vi "InitializeLineDigital.vi"(2 "Store Data":bool, 3 "Image Settings":T1={"Start Position (µm)"={"x"=0.0, "y"=0.0, "z"=0.0}, "End Position (µm)"={"x"=10.0, "y"=10.0, "z"=0.0}, "Image Resolution (nm/pixel)"={"x"=50.0, "y"=50.0, "z"=100.0}, "Image Size (µm)"={"x"=10.0, "y"=10.0, "z"=0.0}, "Image Size (pixel)"={"x"=50, "y"=50, "z"=0}, "Time Resolution\n(ms/pixel)"=7.0, "1st Axis"=0, "2nd Axis"=1, "Retrace"=FALSE, "Estimated Time"=""} {"2nd Axis" items=["x", "y", "z"]; "1st Axis" items=["x", "y", "z"]; "Time Resolution\n(ms/pixel)" format="%.2f"; "Image Resolution (nm/pixel)"."z" format="%.2f"; "Image Resolution (nm/pixel)"."y" format="%.2f"; "Image Resolution (nm/pixel)"."x" format="%.2f"; "Image Size (µm)"."z" format="%.2f"; "Image Size (µm)"."y" format="%.2f"; "Image Size (µm)"."x" format="%.2f"; "End Position (µm)"."z" format="%.2f"; "End Position (µm)"."y" format="%.2f"; "End Position (µm)"."x" format="%.2f"; "Start Position (µm)"."z" format="%.2f"; "Start Position (µm)"."y" format="%.2f"; "Start Position (µm)"."x" format="%.2f"}, 4 "error in (no error)":errorcluster, 5 "Destination:":path) -> (0 "error out":errorcluster, 1 "Busy":bool)   [LabVIEW 2009]
uses:
  ImageSettings.ctt
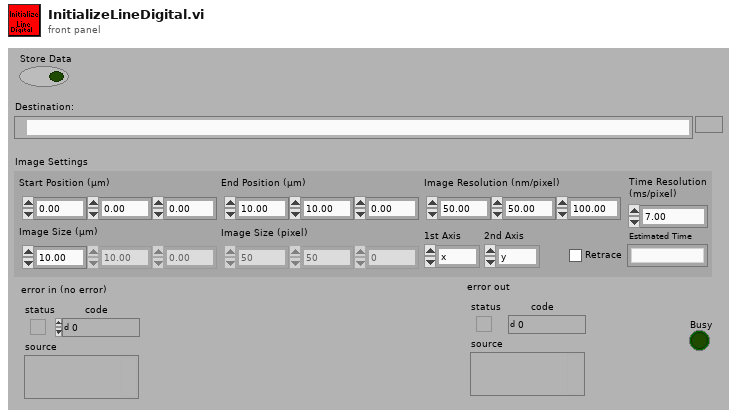
[diagram p1: front panel]
types:
  T1 = typedef "ImageSettings.ctt" = cluster{"Start Position (µm)":cluster{"x":dbl, "y":dbl, "z":dbl}, "End Position (µm)":cluster{"x":dbl, "y":dbl, "z":dbl}, "Image Resolution (nm/pixel)":cluster{"x":dbl, "y":dbl, "z":dbl}, "Image Size (µm)":cluster{"x":dbl, "y":dbl, "z":dbl}, "Image Size (pixel)":cluster{"x":u32, "y":u32, "z":u32}, "Time Resolution\n(ms/pixel)":dbl, "1st Axis":u16, "2nd Axis":u16, "Retrace":bool, "Estimated Time":string}
  T2 = typedef "LineScanStatus.ctt" = cluster{"in line":bool, "line status":cluster{"count":u32, "current":cluster{"x":u32, "y":u32, "z":u32}}, "plane status":cluster{"count":u32, "current":cluster{"x":u32, "y":u32, "z":u32}}, "new line step":cluster{"x":dbl, "y":dbl, "z":dbl}, "new plane step":cluster{"x":dbl, "y":dbl, "z":dbl}}
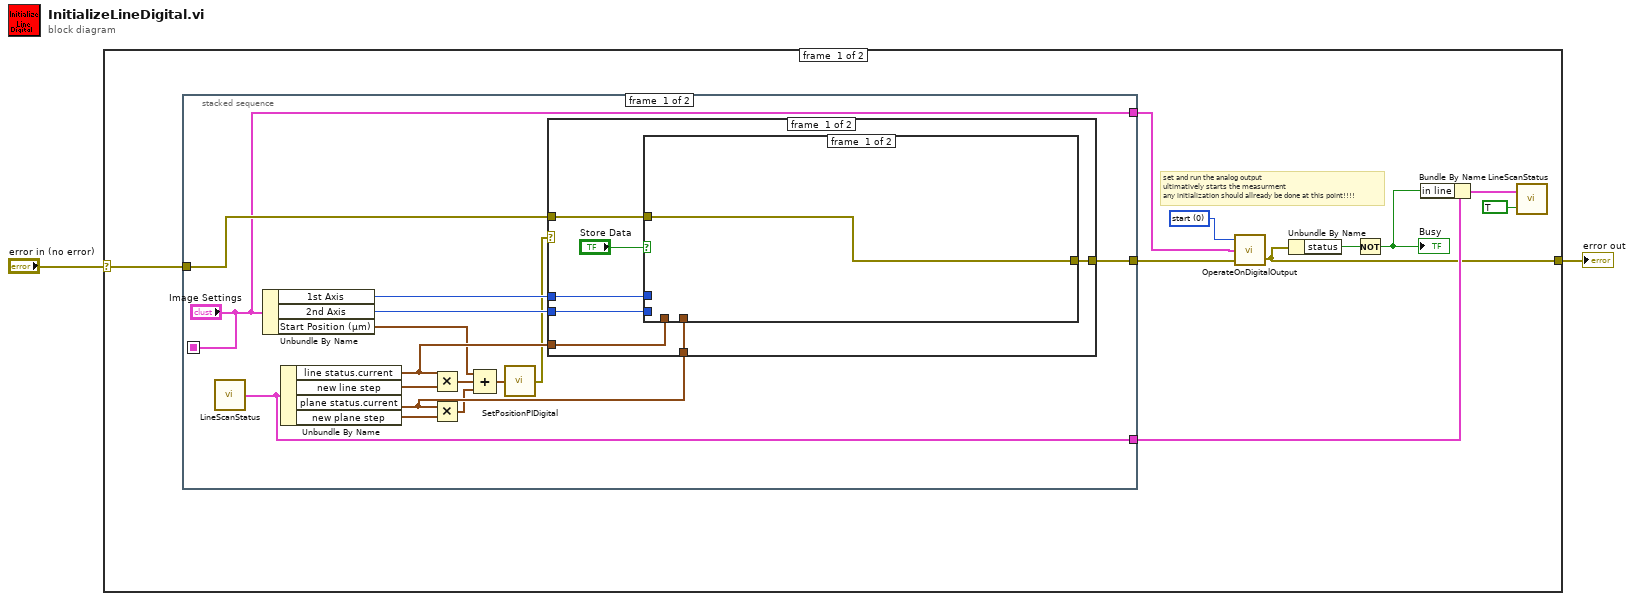
[diagram p0: block diagram]
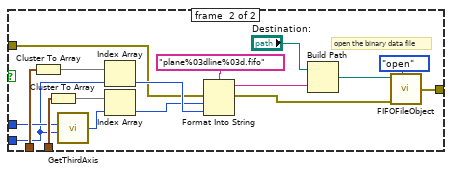
[diagram p2: hidden frame]
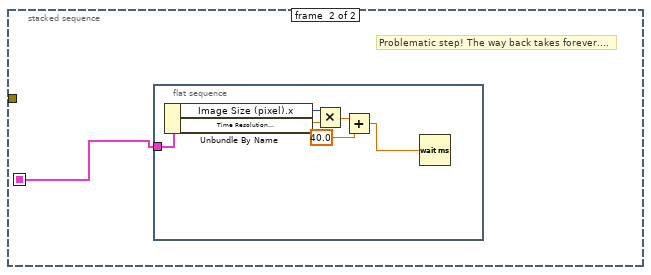
[diagram p4: hidden frame]
diagram:
  n1 = case shown="No Error" "error in (no error)" {
    selector: "error in (no error)" -> [w8 w61]
    tunnel: [w6 w61] -> w2
    frame #0 {
      w4 = u16 0 items=["start", "state", "abort"] ("operation")
      # "set and run the analog output\nultimatively starts the measurment\nany initialization should allready be done at this point!!!!"
      n2 = stacked-sequence {
        seq-local: ["Image Settings" _] -> [_ w54]
        tunnel: [w23 _] -> w10
        tunnel: w8 -> [w22 _]
        tunnel: [w17 _] -> w5
        tunnel: ["Image Settings" _] -> w3
        frame #0 {
          n3 = call "LineScanStatus.vi"() -> ("Linescan Status (output)"=w23:T2)  [unwired: 2 in]
          n4 = Unbundle By Name("Image Settings") -> ("1st Axis"=w21:u16, "2nd Axis"=w20:u16, "Start Position (µm)"=w14:cluster{"x":dbl, "y":dbl, "z":dbl})
          n5 = Unbundle By Name(w23) -> ("line status.current"=w25:cluster{"x":u32, "y":u32, "z":u32}, "new line step"=w27:cluster{"x":dbl, "y":dbl, "z":dbl}, "plane status.current"=w24:cluster{"x":u32, "y":u32, "z":u32}, "new plane step"=w26:cluster{"x":dbl, "y":dbl, "z":dbl})
          n6 = Multiply(x=w25, y=w27) -> (x*y=w19:cluster{"x":dbl, "y":dbl, "z":dbl})
          n7 = Multiply(x=w24, y=w26) -> (x*y=w18:cluster{"x":dbl, "y":dbl, "z":dbl})
          n8 = Compound Arithmetic op=ADD(w14, w19, w18) -> (w16:cluster{"x":dbl, "y":dbl, "z":dbl})
          n9 = call "SetPositionPIDigital.vi"("Current Position (µm)"=w16) -> ("error out"=w15:errorcluster)
          n10 = case shown="No Error" w15 {
            selector: w15 -> [_ w53]
            tunnel: w25 -> [w34 _]
            tunnel: w24 -> [w33 _]
            tunnel: w22 -> [w32 _]
            tunnel: w21 -> [w31 _]
            tunnel: w20 -> [w30 _]
            tunnel: [w29 w53] -> w17
            frame #0 {
              n11 = case shown="True" "Store Data" {
                tunnel: w34 -> [_ w52]
                tunnel: w33 -> [_ w51]
                tunnel: w32 -> [w35 w45]
                tunnel: w31 -> [_ w44]
                tunnel: w30 -> [_ w43]
                tunnel: [w35 w36] -> w29
                frame #0 {
                }
                frame #1 {
                  # "open the binary data file"
                  n12 = Cluster To Array(cluster=w52) -> (array=w48:u32[])
                  n13 = Cluster To Array(cluster=w51) -> (array=w47:u32[])
                  n14 = call "GetThirdAxis.vi"("1st Axis"=w43, "2nd Axis"=w44) -> ("3rd Axis"=w46:i32)  [unwired: 2 in]
                  n15 = Index Array(array=w48, index=w43) -> (element=w50:u32)
                  n16 = Index Array(array=w47, index=w46) -> (element=w49:u32)
                  n17 = Format Into String(format string="plane%03dline%03d.fifo", error in=w45, w49, w50) -> (resulting string=w41:string, error out=w37:errorcluster)  [unwired: 1 in]
                  n18 = Build Path(base path="Destination:", name or relative path=w41) -> (appended path=w42:path)
                  n19 = call "FIFOFileObject.vi"("function (open:0)"=enum16{"open", "write", "close"}."open", "error in (no error)"=w37, "Destination:"=w42) -> ("error out"=w36:errorcluster)  [unwired: 3 in]
                }
              }
            }
            frame #1 {
            }
          }
        }
        frame #1 {
          # "Problematic step! The way back takes forever...."
          n20 = flat-sequence {
            tunnel: w54 -> [w60]
            frame #0 {
              n21 = Unbundle By Name(w60) -> ("Image Size (pixel).x"=w59:u32, "Time Resolution\n(ms/pixel)"=w58:dbl)
              n22 = Multiply(x=w59, y=w58) -> (x*y=w57:dbl)
              n23 = Add(x=w57, y=40.0) -> (x+y=w55:dbl)
              n24 = Wait (ms)(milliseconds to wait=w55) -> ()  [unwired: 1 out]
            }
          }
        }
      }
      n25 = call "OperateOnDigitalOutput.vi"("error in (no error)"=w5, "Image Settings"=w3, "operation"=w4) -> ("error out"=w6:errorcluster)  [unwired: 1 in]
      n26 = Unbundle By Name(w6) -> ("status"=w7:bool)
      n27 = Not(x=w7) -> (.not. x?=w9:bool)
      "Busy" <- w9
      n28 = Bundle By Name(cluster=w10, "in line"=w9) -> (w11:T2)
      n29 = call "LineScanStatus.vi"("Get/Set"=TRUE, "Linescan Status (input)"=w11) -> ()  [unwired: 1 out]
    }
    frame #1 {
    }
  }
  "error out" <- w2
